vi "Main.vi"() -> ()   [LabVIEW 2012]
uses:
  Consumer Message.ctl
  <vilib>/ErrorRing/Error Ring.xnode
  <vilib>/Utility/error.llb/Error Cluster From Error Code.vi
panel:
  in  "Producer Error":bool
  in  "Consumer Error":bool
  out "Consumer Shutdown?":bool
  out "State to Execute":string
  out "High Priority?":bool
  out "Backlog":u8(slide) scale=0.0..100.0
  out "Processed Value":i32
  in  "High Priority Message":bool
  in  "Normal Priority Message":bool
  in  "Stop":bool
  # "Number of enqueued\nmessages waiting to\nbe processed"
  # "Current data being\nprocessed in consumer loop"
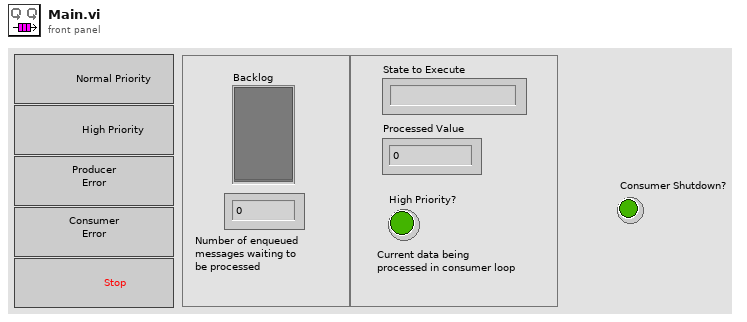
[diagram p1: front panel]
types:
  T1 = typedef "Consumer Message.ctl" = cluster{"Consumer State":string, "Boolean Data":bool, "Numeric Data":i32, "Error":errorcluster}
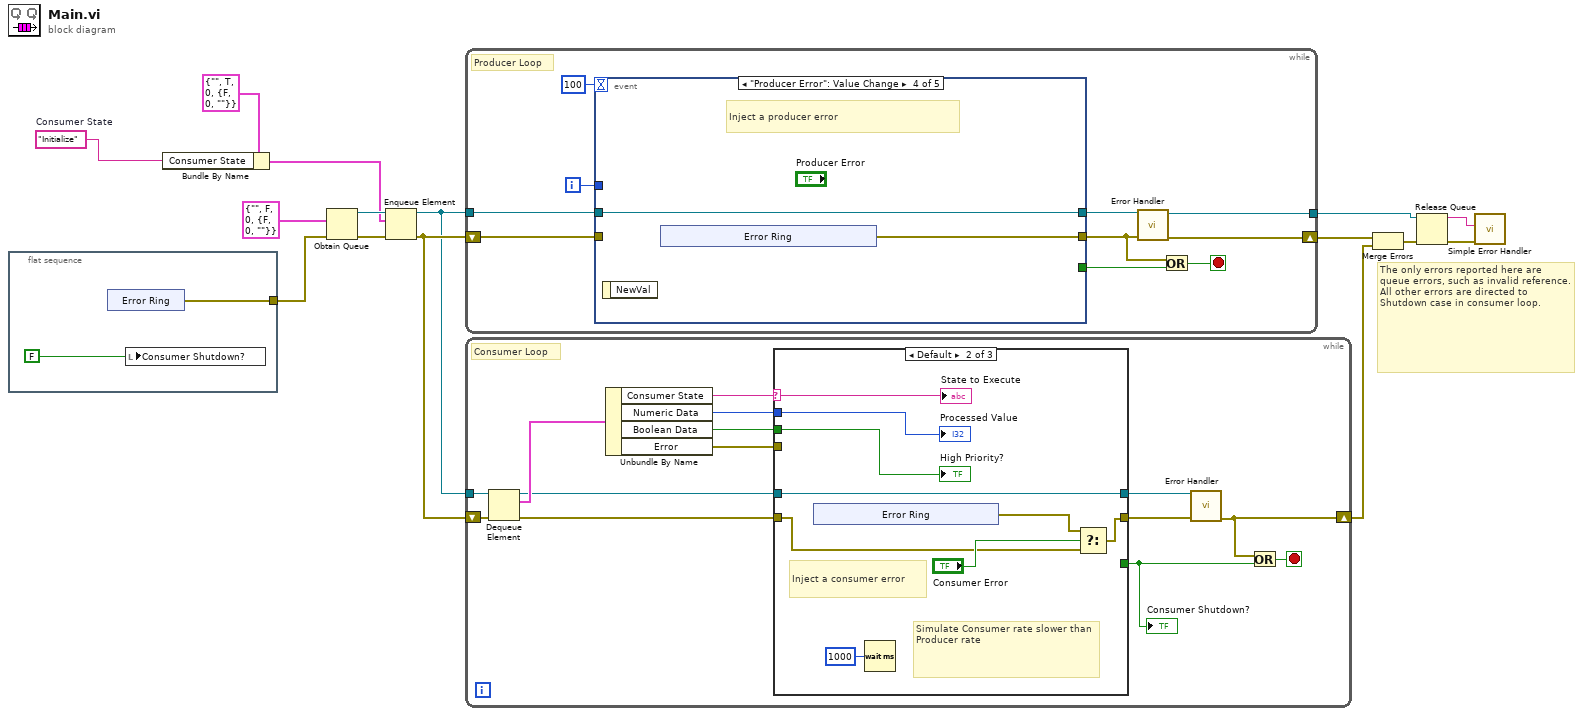
[diagram p0: block diagram]
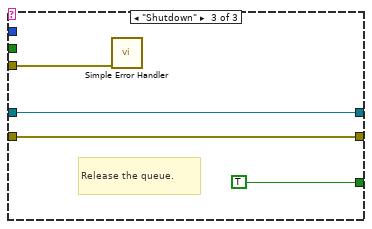
[diagram p3: hidden frame]
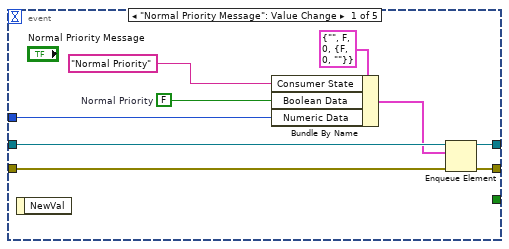
[diagram p4: hidden frame]
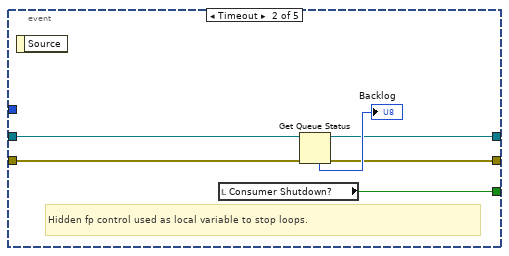
[diagram p5: hidden frame]
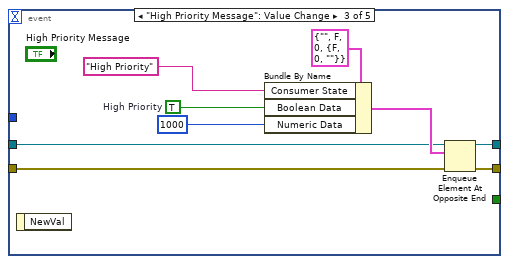
[diagram p6: hidden frame]
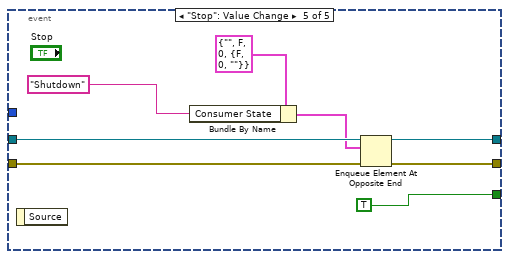
[diagram p7: hidden frame]
diagram:
  w8 = "Initialize"  # Consumer State
  # "The only errors reported here are queue errors, such as invalid reference.  All other errors are directed to Shutdown case in consumer loop."
  n1 = flat-sequence {
    tunnel: [w16] -> w10
    frame #0 {
      n2 = xnode "Error Ring"() -> ("error out"=w16:errorcluster)
      n3 = local write "Consumer Shutdown?"(FALSE ("Stop Loops (local)")) -> ()
    }
  }
  n4 = Bundle By Name(cluster=T1 {"Consumer State"="", "Boolean Data"=TRUE, "Numeric Data"=0, "Error"={"status"=FALSE, "code"=0, "source"=""}} ("Consumer Message"), "Consumer State"=w8) -> (w9:T1)
  n5 = Obtain Queue(element data type=T1 {"Consumer State"="", "Boolean Data"=FALSE, "Numeric Data"=0, "Error"={"status"=FALSE, "code"=0, "source"=""}}, error in (no error)=w10) -> (queue out=w12:refnum<queue>, error out=w15:errorcluster)  [unwired: 3 in, 1 out]
  n6 = Enqueue Element(queue=w12, element=w9, error in (no error)=w15) -> (queue out=w11:refnum<queue>, error out=w13:errorcluster)  [unwired: 1 in, 1 out]
  n7 = while {
    tunnel: w11 -> [w28]
    shift-right: [w20] -> w6
    shift-left: w13 -> [w27]
    tunnel: [w19] -> w2
    i -> [w26]
    stop <- w22 stop-if-true
    # "Producer Loop"
    n8 = event shown="[3] \"Producer Error\": Value Change" {
      selector: _ -> [_ _ _ _ _]
      dyn-events: _ -> [_ _ _ _ _]
      timeout: 100 -> [_ _ _ _ _]
      tunnel: w28 -> [w37 w41 w44 w53 w66]
      tunnel: w27 -> [w35 w40 w51 _ w64]
      tunnel: [w36 w39 w52 w54 w63] -> w21
      tunnel: [_ w43 _ _ TRUE] -> w23
      tunnel: w26 -> [w34 _ _ _ _]
      tunnel: [w30 w38 w47 w53 w62] -> w25
      event "Normal Priority Message": Value Change {
        w31 = FALSE  # Normal Priority
        n9 = event-data() -> ()  [unwired: 1 in, 1 out]
        n10 = Bundle By Name(cluster=T1 {"Consumer State"="", "Boolean Data"=FALSE, "Numeric Data"=0, "Error"={"status"=FALSE, "code"=0, "source"=""}}, "Consumer State"="Normal Priority" ("String Data"), "Boolean Data"=w31, "Numeric Data"=w34) -> (w33:T1)
        n11 = Enqueue Element(queue=w37, element=w33, error in (no error)=w35) -> (queue out=w30:refnum<queue>, error out=w36:errorcluster)  [unwired: 1 in, 1 out]
      }
      event Timeout {
        # "Hidden fp control used as local variable to stop loops."
        n12 = event-data() -> ()  [unwired: 1 in, 1 out]
        n13 = local read "Consumer Shutdown?"() -> (w43:bool)
        n14 = Get Queue Status(queue=w41, error in (no error)=w40) -> (queue out=w38:refnum<queue>, error out=w39:errorcluster, # elements in queue=→"Backlog":i32)  [unwired: 1 in, 5 out]
      }
      event "High Priority Message": Value Change {
        w46 = TRUE  # High Priority
        n15 = event-data() -> ()  [unwired: 1 in, 1 out]
        n16 = Bundle By Name(cluster=T1 {"Consumer State"="", "Boolean Data"=FALSE, "Numeric Data"=0, "Error"={"status"=FALSE, "code"=0, "source"=""}}, "Consumer State"="High Priority" ("String Data"), "Boolean Data"=w46, "Numeric Data"=1000) -> (w49:T1)
        n17 = Enqueue Element At Opposite End(queue=w44, element=w49, error in (no error)=w51) -> (queue out=w47:refnum<queue>, error out=w52:errorcluster)  [unwired: 1 in, 1 out]
      }
      event "Producer Error": Value Change {
        # "Inject a producer error"
        n18 = event-data() -> ()  [unwired: 1 in, 1 out]
        n19 = xnode "Error Ring"() -> ("error out"=w54:errorcluster)
      }
      event "Stop": Value Change {
        n20 = event-data() -> ()  [unwired: 1 in, 1 out]
        n21 = Bundle By Name(cluster=T1 {"Consumer State"="", "Boolean Data"=FALSE, "Numeric Data"=0, "Error"={"status"=FALSE, "code"=0, "source"=""}}, "Consumer State"="Shutdown") -> (w59:T1)
        n22 = Enqueue Element At Opposite End(queue=w66, element=w59, error in (no error)=w64) -> (queue out=w62:refnum<queue>, error out=w63:errorcluster)  [unwired: 1 in, 1 out]
      }
    }
    n23 = call "Error Handler.vi"("error in"=w21, "queue in"=w25) -> ("error out"=w20:errorcluster, "queue out"=w19:refnum<queue>)  [unwired: 8 in]
    n24 = Or(x=w21, y=w23) -> (x .or. y?=w22:bool)
  }
  n25 = while {
    tunnel: w11 -> [w80]
    shift-right: [w69] -> w7
    shift-left: w13 -> [w79]
    stop <- w70 stop-if-true
    # "Consumer Loop"
    n26 = Dequeue Element(queue=w80, error in (no error)=w79) -> (queue out=w68:refnum<queue>, element=w78:T1, error out=w67:errorcluster)  [unwired: 1 in, 1 out]
    n27 = Unbundle By Name(w78) -> ("Consumer State"=w77:string, "Numeric Data"=w76:i32, "Boolean Data"=w75:bool, "Error"=w72:errorcluster)
    n28 = case shown="Default" w77 {
      selector: w77 -> [_ w88 _]
      tunnel: [_ _ TRUE] -> w71
      tunnel: w67 -> [w81 w84 w97]
      tunnel: [w81 w85 w97] -> w74
      tunnel: w76 -> [_ w91 _]
      tunnel: w75 -> [_ w90 _]
      tunnel: w68 -> [w82 w89 w98]
      tunnel: [w82 w89 w98] -> w73
      tunnel: w72 -> [_ _ w99]
      frame "Initialize" {
      }
      frame Default {
        # "Inject a consumer error"
        # "Simulate Consumer rate slower than Producer rate"
        n29 = xnode "Error Ring"() -> ("error out"=w83:errorcluster)
        n30 = Wait (ms)(milliseconds to wait=u32 1000) -> ()  [unwired: 1 out]
        n31 = Select(t=w83, s="Consumer Error", f=w84) -> (s? t:f=w85:errorcluster)
        "Processed Value" <- w91
        "High Priority?" <- w90
        "State to Execute" <- w88
      }
      frame "Shutdown" {
        # "Release the queue."
        n32 = call <vilib>:"Simple Error Handler.vi"("error in (no error)"=w99) -> ()  [unwired: 4 in, 5 out]
      }
    }
    "Consumer Shutdown?" <- w71
    n33 = call "Error Handler.vi"("error in"=w74, "queue in"=w73) -> ("error out"=w69:errorcluster)  [unwired: 8 in, 1 out]
    n34 = Or(x=w69, y=w71) -> (x .or. y?=w70:bool)
  }
  n35 = Merge Errors(w6, w7) -> (w3:errorcluster)
  n36 = Release Queue(queue=w2, error in (no error)=w3) -> (queue name=w5:string, error out=w4:errorcluster)  [unwired: 1 in, 1 out]
  n37 = call <vilib>:"Simple Error Handler.vi"("error source (\" \")"=w5, "error in (no error)"=w4) -> ()  [unwired: 3 in, 5 out]
